vi "Set Output State.vi"(8 "error in (no error)":errorcluster, 10 "Output State":bool, 11 "Cooler in":refnum<class "Cooler.lvclass">) -> (0 "error out":errorcluster, 3 "Cooler out":refnum<class "Cooler.lvclass">)   [LabVIEW 2012, in "Cooler.lvlib" / "Cooler.lvclass"]
uses:
  Cooler.lvclass
  Cooler.lvclass/Cooler.ctl
  Cooler UI/Update Pump Msg/Update Pump Msg.lvclass/Update Pump Msg.ctl
  <vilib>/ActorFramework/Message Enqueuer/Message Enqueuer.lvclass/Message Enqueuer.ctl
  <vilib>/ActorFramework/Time-Delayed Send Message/Time-Delay Override Options.ctl
  Dual Controller/Power On Msg/Power On Msg.lvclass
  <vilib>/ActorFramework/Message Enqueuer/Enqueue.vi
  Simulation/Simulation Data_Global.vi
  <vilib>/ActorFramework/Message Priority Queue/Priority Enqueue.vi
  Cooler UI/Update Pump Msg/Update Pump Msg.lvclass
  Dual Controller/Power Off Msg/Power Off Msg.lvclass
  Simulation/Simulation.lvlib
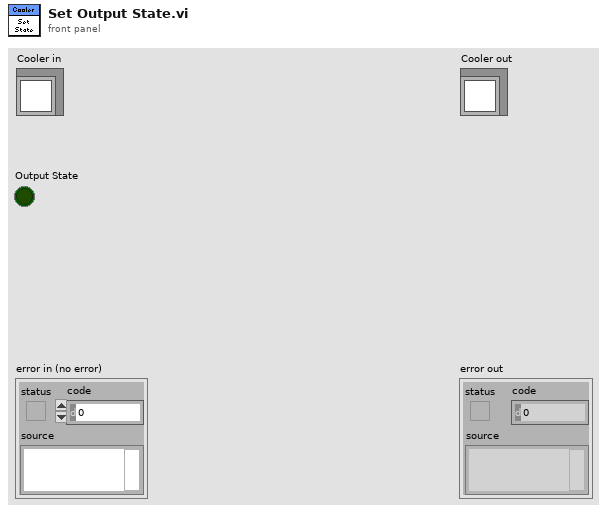
[diagram p1: front panel]
types:
  T1 = typedef "Time-Delay Override Options.ctl" = enum16{"Send next copy now", "Skip next scheduled copy", "Send next copy now and stop all further copies", "Stop all further copies"}
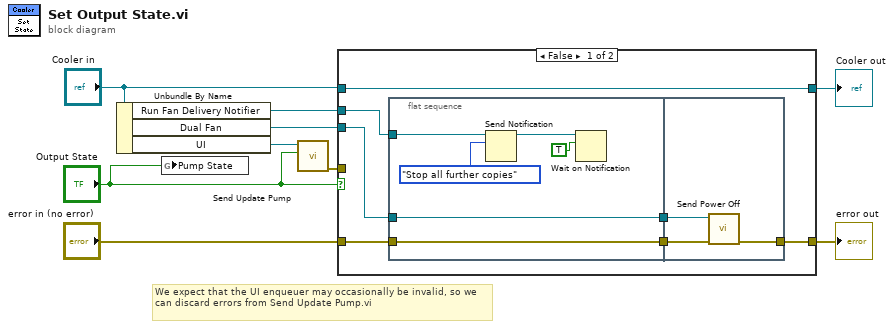
[diagram p0: block diagram]
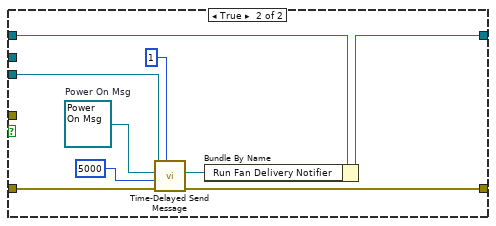
[diagram p2: hidden frame]
diagram:
  # "We expect that the UI enqueuer may occasionally be invalid, so we can discard errors from Send Update Pump.vi"
  n1 = Unbundle By Name("Cooler in") -> ("Run Fan Delivery Notifier"=w5:refnum<notifier>, "Dual Fan"=w9:refnum<class "Message Enqueuer.lvclass">, "UI"=w3:refnum<class "Message Enqueuer.lvclass">)
  n2 = global write "Simulation Data_Global.vi" "Pump State"("Output State") -> ()
  n3 = call "Send Update Pump.vi"("Output State"="Output State", "enqueuer"=w3) -> ("error out"=w1:errorcluster)  [unwired: 9 in]
  n4 = case shown="False" "Output State" {
    tunnel: "error in (no error)" -> [w13 w34]
    tunnel: w9 -> [w10 w32]
    tunnel: [w12 w33] -> w8
    tunnel: "Cooler in" -> [w16 w27]
    tunnel: [w16 w26] -> w6
    tunnel: w5 -> [w15 _]
    tunnel: w1 -> [_ _]
    frame False {
      n5 = flat-sequence {
        tunnel: w15 -> [w22]
        tunnel: [w19] -> w14
        tunnel: w13 -> [w19]
        tunnel: [w18] -> w11
        tunnel: w10 -> [w18]
        tunnel: w14 -> [w25]
        tunnel: [w24] -> w12
        tunnel: w11 -> [w23]
        frame #0 {
          n6 = Send Notification(notification=Time-Delay_Override_Options."Stop all further copies", notifier=w22) -> (notifier out=w20:refnum<notifier>)  [unwired: 1 in, 1 out]
          n7 = Wait on Notification(notifier=w20, ignore previous (F)=TRUE) -> ()  [unwired: 2 in, 4 out]
        }
        frame #1 {
          n8 = call "Send Power Off.vi"("error in (no error)"=w25, "enqueuer"=w23) -> ("error out"=w24:errorcluster)  [unwired: 9 in]
        }
      }
    }
    frame True {
      w31 = refnum<class "Power On Msg.lvclass"> refnum  # Power On Msg
      n9 = call <vilib>:"Time-Delayed Send Message.vi"("# Copies (0 = infinite repeat)"=u32 1, "error in (no error)"=w34, "Milliseconds To Wait"=5000, "Message"=w31, "Message Enqueuer"=w32) -> ("error out"=w33:errorcluster, "Delivery Notifier"=w29:refnum<notifier>)  [unwired: 5 in]
      n10 = Bundle By Name(cluster=w27, "Run Fan Delivery Notifier"=w29) -> (w26:refnum<class "Cooler.lvclass">)
    }
  }
  "error out" <- w8
  "Cooler out" <- w6
